vi "ReadInputTunnels.vi"(9 "Structure in":refnum<class "Structure.lvclass">) -> (3 "Structure out":refnum<class "Structure.lvclass">, 4 "tunnels":refnum<class "Tunnel.lvclass">[](array[class]))   [LabVIEW 2014, in "Raspberry Pi Compatible Compiler for LabVIEW.lvlib" / "Structure.lvclass"]
uses:
  Structure.lvclass
  Tunnel/Tunnel.lvclass
  Structure.lvclass/Structure.ctl
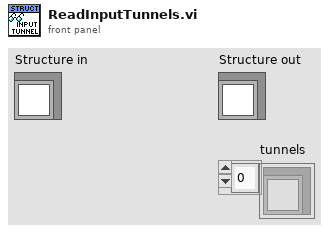
[diagram p1: front panel]
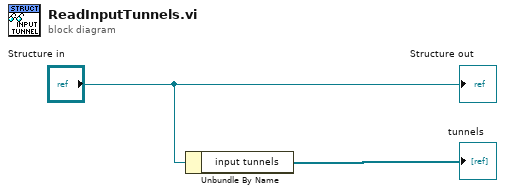
[diagram p0: block diagram]
diagram:
  n1 = Unbundle By Name("Structure in") -> ("input tunnels"=→"tunnels":refnum<class "Tunnel.lvclass">[])
  "Structure out" <- "Structure in"
